vi "CLD 10 CSV file utility.vi"(8 "Error In":errorcluster, 10 "[Data In]":T1[](array[typedef]), 11 "CSV File Enum":T2) -> (0 "Error Out":errorcluster, 3 "[Data Out]":T1[](array[typedef]))   [LabVIEW 2019]
doc: "This VI is an FGV that reads the \"CLD CSV File.csv\" file and places the data into the \"CLD 10 CSV file data structure.ctl\" data cluster.\n\nTesting Tip:\n\nThere is a Boolean control that can be defaulted to insure the FGV looks for the data file either in the same directory as the FGV (useful for testing) or in the callers directory, if the caller is in a standard CLD test hierarchy, one directory above the subVI directory."
uses:
  CLD 10 CSV file enum.ctl
  CLD 10 CSV file data structure.ctl
  <vilib>/Utility/file.llb/Read Delimited Spreadsheet (string).vi
  <vilib>/Utility/file.llb/Write To Spreadsheet File (string).vi
panel:
  in  "(T) Main (F) SubVI":bool=TRUE
  # "Default T,   Used for Testing only"
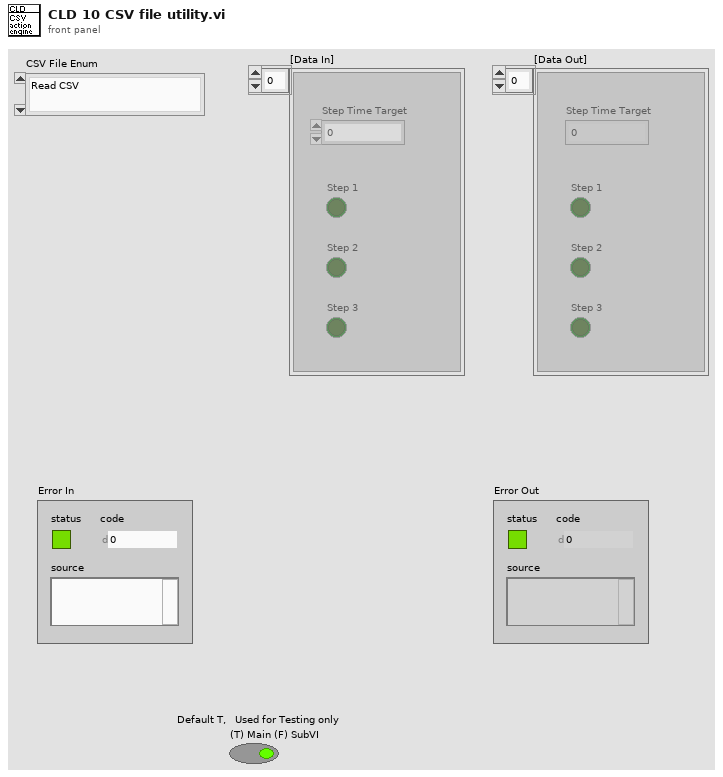
[diagram p1: front panel]
types:
  T1 = typedef "CLD 10 CSV file data structure.ctl" = cluster{"Step Time Target":i32, "Step 1":bool, "Step 2":bool, "Step 3":bool}
  T2 = typedef "CLD 10 CSV file enum.ctl" = enum16{"Read CSV", "Write CSV"}
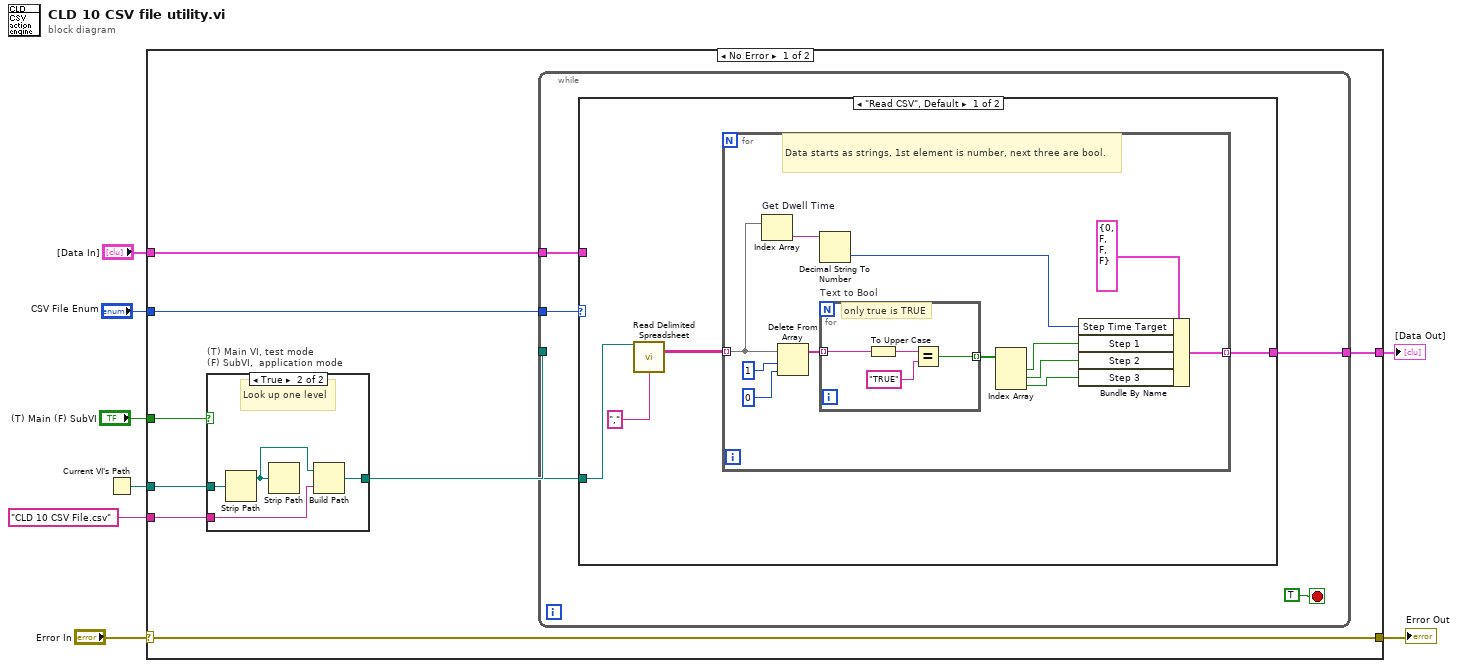
[diagram p0: block diagram]
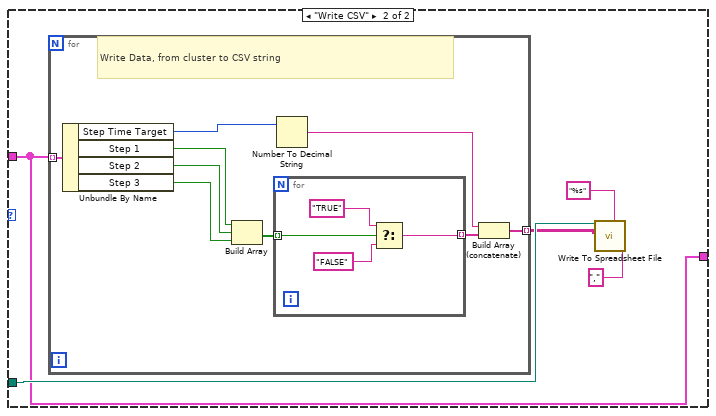
[diagram p2: hidden frame]
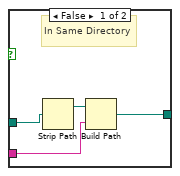
[diagram p3: hidden frame]
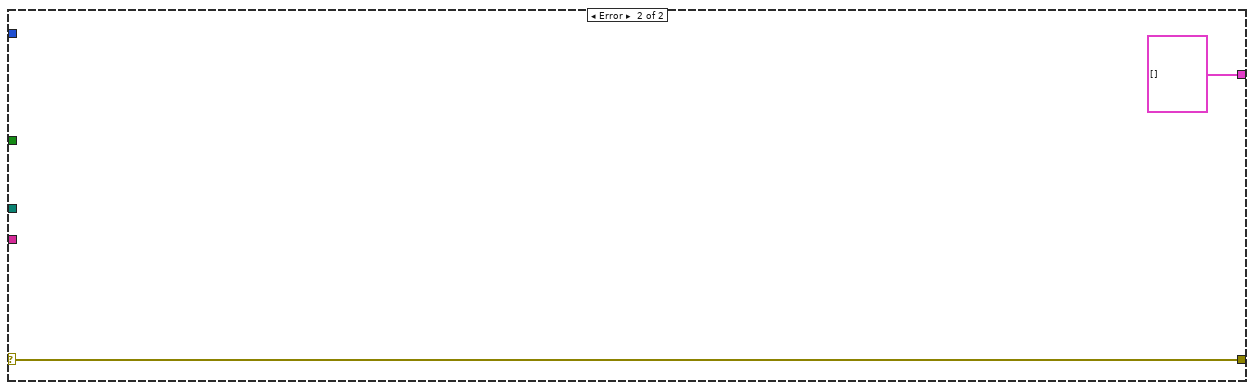
[diagram p4: hidden frame]
diagram:
  n1 = Current VI's Path() -> (path=w5:path)
  n2 = case shown="No Error" "Error In" {
    selector: "Error In" -> [w9 w69]
    tunnel: [w16 T1[] [] ("[Data In]")] -> w8
    tunnel: "(T) Main (F) SubVI" -> [w15 _]
    tunnel: "CLD 10 CSV File.csv" -> [w14 _]
    tunnel: w5 -> [w13 _]
    tunnel: "CSV File Enum" -> [w11 _]
    tunnel: "[Data In]" -> [w10 _]
    tunnel: [w9 w69] -> w1
    frame No Error {
      n3 = case "(T) Main VI, test mode\n(F) SubVI,  application mode" shown="True" w15 {
        tunnel: w14 -> [w61 w66]
        tunnel: w13 -> [w62 w67]
        tunnel: [w60 w65] -> w12
        frame False {
          # "In Same Directory"
          n4 = Strip Path(path=w62) -> (stripped path=w63:path)  [unwired: 1 out]
          n5 = Build Path(base path=w63, name or relative path=w61) -> (appended path=w60:path)
        }
        frame True {
          # "Look up one level"
          n6 = Strip Path(path=w67) -> (stripped path=w64:path)  [unwired: 1 out]
          n7 = Strip Path(path=w64) -> ()  [unwired: 2 out]
          n8 = Build Path(base path=w64, name or relative path=w66) -> (appended path=w65:path)
        }
      }
      n9 = while {
        tunnel: w12 -> [w19]
        tunnel: w11 -> [w20]
        tunnel: [w18] -> w16
        tunnel: w10 -> [w17]
        stop <- TRUE stop-if-true
        n10 = case shown="\"Read CSV\", Default" w20 {
          tunnel: w19 -> [w24 w46]
          tunnel: [w25 w42] -> w18
          tunnel: w17 -> [_ w42]
          frame "Read CSV", Default {
            n11 = call-poly <vilib>:"Read Delimited Spreadsheet.vi"("file path (dialog if empty)"=w24, "delimiter (\\t)"="," ("delimiter (\\t)")) -> ("all rows"=w23:string[][])  [unwired: 8 in, 5 out]
            n12 = for {
              tunnel: w23 -> [w34] mode=indexing
              tunnel: [w37] -> w25 mode=indexing
              # "Data starts as strings, 1st element is number, next three are bool."
              n13 = Index Array "Get Dwell Time"(array=w34) -> (element=w36:string)  [unwired: 1 in]
              n14 = Delete From Array(array=w34, length=1, index=0) -> (array with subset deleted=w27:string[])  [unwired: 1 out]
              n15 = Decimal String To Number(string=w36) -> (number=w35:i32)  [unwired: 2 in, 1 out]
              n16 = for "Text to Bool" {
                tunnel: w27 -> [w41] mode=indexing
                tunnel: [w38] -> w31 mode=indexing
                # "only true is TRUE"
                n17 = To Upper Case(1:w41) -> (0:w40:string)
                n18 = Equal?(x=w40, y="TRUE") -> (x = y?=w38:bool)
              }
              n19 = Index Array(array=w31) -> (element #1=w30:bool, element #2=w29:bool, element #3=w28:bool)  [unwired: 3 in]
              n20 = Bundle By Name(cluster=T1 {"Step Time Target"=0, "Step 1"=FALSE, "Step 2"=FALSE, "Step 3"=FALSE} ("CSV File Data Structure"), "Step Time Target"=w35, "Step 1"=w30, "Step 2"=w29, "Step 3"=w28) -> (w37:T1)
            }
          }
          frame "Write CSV" {
            n21 = for {
              tunnel: w42 -> [w55] mode=indexing
              tunnel: [w47] -> w44 mode=indexing
              # "Write Data, from cluster to CSV string"
              n22 = Unbundle By Name(w55) -> ("Step Time Target"=w54:i32, "Step 1"=w53:bool, "Step 2"=w52:bool, "Step 3"=w51:bool)
              n23 = Build Array(w53, w52, w51) -> (w50:bool[])
              n24 = for {
                tunnel: w50 -> [w59] mode=indexing
                tunnel: [w56] -> w48 mode=indexing
                n25 = Select(t="TRUE", s=w59, f="FALSE") -> (s? t:f=w56:string)
              }
              n26 = Number To Decimal String(number=w54) -> (decimal integer string=w49:string)  [unwired: 1 in]
              n27 = Build Array (concatenate)(w49, w48) -> (w47:string[])
            }
            n28 = call-poly <vilib>:"Write To Spreadsheet File.vi"("delimiter (\\t)"="," ("delimiter (\\t)"), "format (%s)"="%s", "2D data"=w44, "file path (dialog if empty)"=w46) -> ()  [unwired: 4 in, 1 out]
          }
        }
      }
    }
    frame Error {
    }
  }
  "[Data Out]" <- w8
  "Error Out" <- w1
